vi "Transient Capture - Fire Shot and Wait.vi"(7 "Soft Trigger":bool=TRUE, 8 "error in":errorcluster, 10 "Carrier Connection In":T1, 11 "AI Connection In":T1) -> (0 "error out":errorcluster, 2 "Carrier Connection Out":T1, 3 "AI Connection Out":T1)   [LabVIEW 2017, in "Communications Library.lvlib"]
doc: "Triggers the transient shot and waits until data is available for download."
uses:
  Communications Library.lvlib
  Typedefs/DTACQ Connection Data--Cluster.ctl
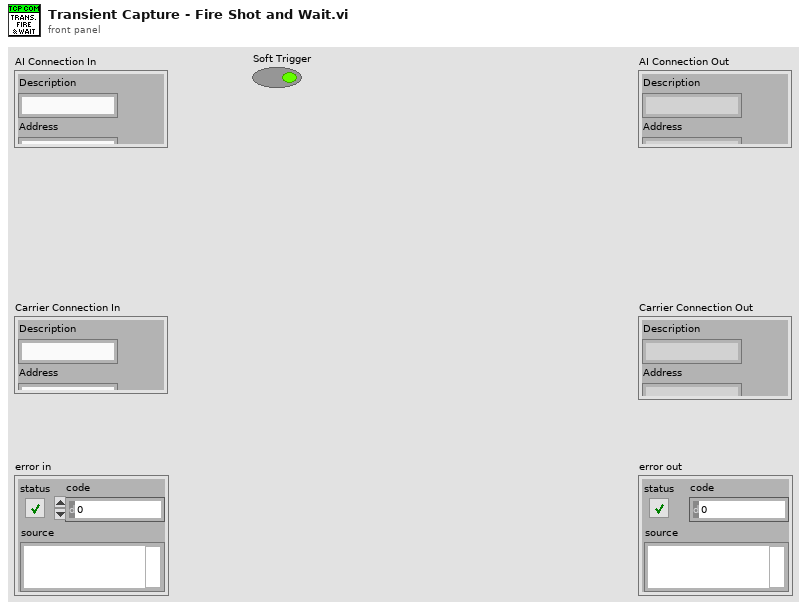
[diagram p1: front panel]
types:
  T1 = typedef "Communications Library.lvlib/DTACQ Connection Data--Cluster.ctl" = cluster{"Description":string, "Address":string, "Port":u16, "timeout (ms)":i32, "Termination Character":string, "TCP Connection Reference":refnum<k5>, "Open Connection":bool}
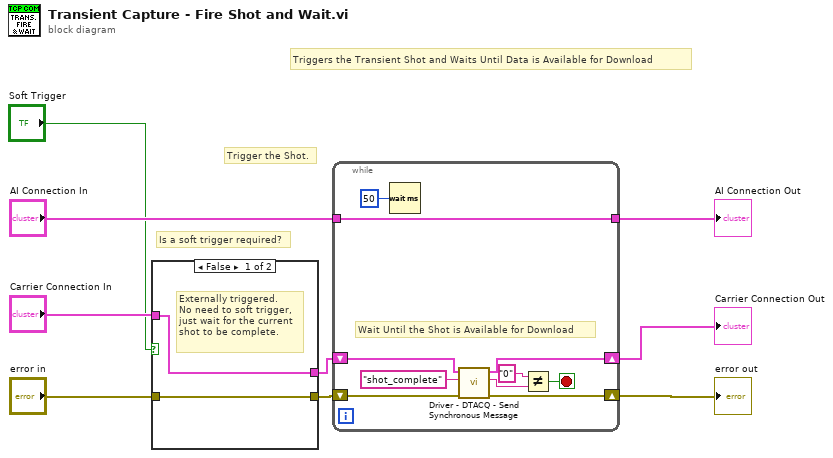
[diagram p0: block diagram]
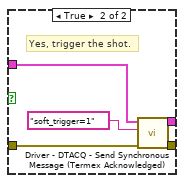
[diagram p2: hidden frame]
diagram:
  # "Is a soft trigger required?"
  # "Triggers the Transient Shot and Waits Until Data is Available for Download"
  # "Trigger the Shot."
  n1 = case shown="False" "Soft Trigger" {
    tunnel: "error in" -> [w11 w15]
    tunnel: [w11 w14] -> w5
    tunnel: "Carrier Connection In" -> [w10 w13]
    tunnel: [w10 w12] -> w3
    frame False {
      # "Externally triggered.\nNo need to soft trigger,\njust wait for the current\nshot to be complete."
    }
    frame True {
      # "Yes, trigger the shot."
      n2 = call "Driver - DTACQ - Send Synchronous Message (Termex Acknowledged).vi"("error in"=w15, "Message to Send"="soft_trigger=1", "DTACQ Connection Data In"=w13) -> ("error out"=w14:errorcluster, "DTACQ Connection Data Out"=w12:T1)  [unwired: 5 in, 2 out]
    }
  }
  n3 = while {
    shift-right: [w22] -> w9
    shift-left: w5 -> [w23]
    shift-right: [w19] -> w8
    shift-left: w3 -> [w18]
    tunnel: "AI Connection In" -> [w17]
    tunnel: [w17] -> w7
    stop <- w21 stop-if-true
    # "Wait Until the Shot is Available for Download"
    n4 = Wait (ms)(milliseconds to wait=u32 50) -> ()  [unwired: 1 out]
    n5 = call "Driver - DTACQ - Send Synchronous Message.vi"("error in"=w23, "Message to Send"="shot_complete", "DTACQ Connection Data In"=w18) -> ("error out"=w22:errorcluster, "Read String"=w24:string, "DTACQ Connection Data Out"=w19:T1)  [unwired: 5 in, 1 out]
    n6 = Not Equal?(x="0" ("y"), y=w24) -> (x != y?=w21:bool)
  }
  "Carrier Connection Out" <- w8
  "error out" <- w9
  "AI Connection Out" <- w7
